vi "Lab7_Spectrum_Analyzer.vi"() -> ()   [LabVIEW 2016]
uses:
  <vilib>/Analysis/4window.llb/windowTd.ctl
  <vilib>/DAQmx/read.llb/DAQmx Read (Analog Wfm 1Chan NSamp).vi
  <vilib>/DAQmx/create/channels.llb/DAQmx Create Channel (AI-Voltage-Basic).vi
  <vilib>/DAQmx/configure/timing.llb/DAQmx Timing (Sample Clock).vi
  <vilib>/DAQmx/miscellaneous.llb/DAQmx Fill In Error Info.vi
  <vilib>/measure/maspectr.llb/FFT Power Spectrum and PSD for 1 Chan.vi
  <vilib>/measure/NI_MAPro.lvlib
  <vilib>/measure/NI_MABase.lvlib
  <vilib>/Analysis/NI_AALPro.lvlib
panel:
  out "quantized signal":waveform(ext)(graph)
  in  "full scale":dbl
  in  "number of bits":i16
  out "RMS dBV":dbl
  out "RMS":dbl
  out "Peak to Peak":dbl
  in  "rate":dbl=1000.0 format="%0.2f"
  out "Signal":waveform(dbl)(graph)
  in  "averaging parameters":T1={"averaging mode"=enum."No averaging", "weighting mode"=enum."Exponential", "number of averages"=10} {"number of averages" min=1}
  in  "dB On (F)":bool
  in  "window":T2=1 items=["Rectangle"=0, "Hanning"=1, "Hamming"=2, "Blackman-Harris"=3, "Exact Blackman"=4, "Blackman"=5, "Flat Top"=6, "4 Term B-Harris "=7, "7 Term B-Harris"=8, "Low Sidelobe"=9, "Blackman Nuttall"=11, "Triangle"=30, "Bartlett-Hanning"=31, "Bohman"=32, "Parzen"=33, "Welch"=34, "Kaiser"=60, "Dolph-Chebyshev"=61, "Gaussian"=62]
  in  "stop":bool
  in  "number of samples per channel":i32=-1
  out "Spectrum":cluster{"f0":dbl, "df":dbl, "magnitude":dbl[]}(graph)
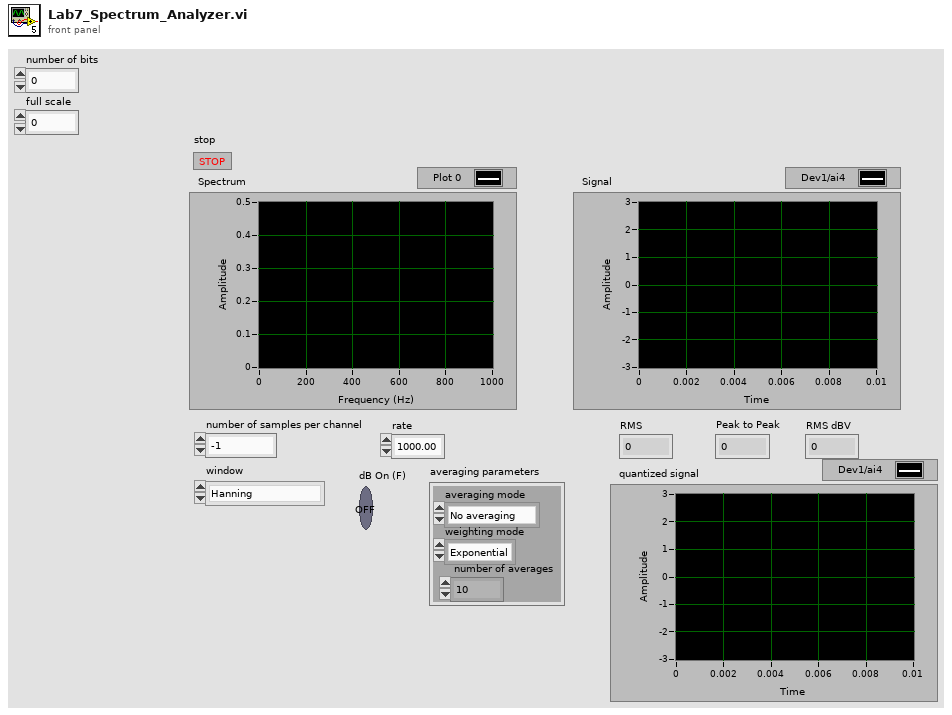
[diagram p1: front panel]
types:
  T1 = cluster{"averaging mode":enum16{"No averaging", "Vector averaging", "RMS averaging", "Peak hold"}, "weighting mode":enum16{"Linear", "Exponential"}, "number of averages":u32}
  T2 = typedef "NI_AALPro.lvlib/windowTd.ctl" = u32
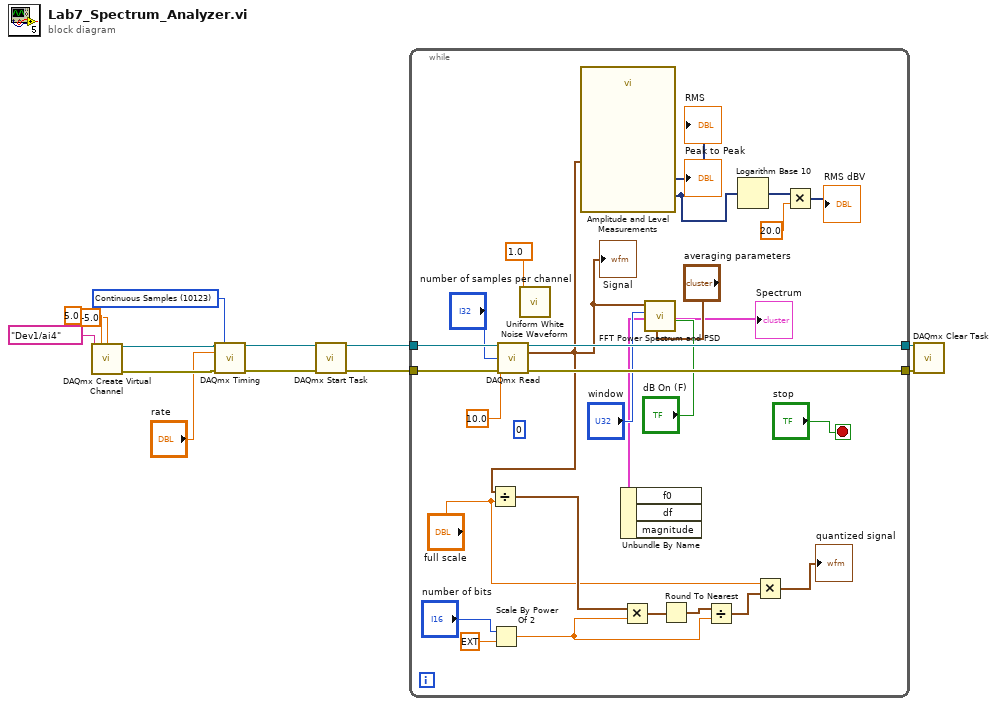
[diagram p0: block diagram]
diagram:
  w9 = 10123 items=["Finite Samples"=10178, "Continuous Samples"=10123, "Hardware Timed Single Point"=12522] ("sample mode")
  n1 = call-poly <vilib>:"DAQmx Create Virtual Channel.vi"("maximum value"=5.0, "minimum value"=-5.0, "physical channels"=tag "Dev1/ai4") -> ("task out"=w10:refnum<k21>, "error out"=w6:errorcluster)  [unwired: 11 in]
  n2 = call-poly <vilib>:"DAQmx Timing.vi"("task/channels in"=w10, "sample mode"=w9, "rate"="rate", "error in"=w6) -> ("task out"=w8:refnum<k21>, "error out"=w5:errorcluster)  [unwired: 10 in]
  n3 = call <vilib>:"DAQmx Start Task.vi"("task/channels in"=w8, "error in"=w5) -> ("task out"=w7:refnum<k21>, "error out"=w4:errorcluster)  [unwired: 12 in]
  n4 = while {
    tunnel: w7 -> [w40]
    tunnel: w4 -> [w37]
    tunnel: [w36] -> w3
    tunnel: [w35] -> w2
    stop <- "stop" stop-if-true
    (unwired) 0 ("seed")
    n5 = Scale By Power Of 2(n="number of bits", x=ext 1.0) -> (x*2^n=w19:ext)
    n6 = call-poly <vilib>:"DAQmx Read.vi"("task/channels in"=w40, "number of samples per channel"="number of samples per channel", "timeout"=10.0, "error in"=w37) -> ("task out"=w36:refnum<k21>, "data"=w22:waveform(dbl), "error out"=w35:errorcluster)  [unwired: 9 in]
    "Signal" <- w22
    n7 = Divide(x=w22, y="full scale") -> (x/y=w21:waveform(dbl))
    n8 = call <vilib>:"Uniform White Noise Waveform.vi"("amplitude"=1.0) -> ()  [unwired: 9 in, 2 out]
    n9 = call "Amplitude and Level Measurements"("Signals"=w22) -> ("RMS"=w29:dynamicdata, "Peak to Peak"=→"Peak to Peak":dynamicdata)  [unwired: 12 in, 1 out]
    "RMS" <- w29
    n10 = Multiply(x=w21, y=w19) -> (x*y=w20:waveform(ext))
    n11 = call-poly <vilib>:"FFT Power Spectrum and PSD.vi"("averaging parameters"="averaging parameters", "dB On (F)"="dB On (F)", "window"="window", "time signal"=w22) -> ("Power Spectrum / PSD"=w24:cluster{"f0":dbl, "df":dbl, "magnitude":dbl[]})  [unwired: 4 in, 3 out]
    "Spectrum" <- w24
    n12 = Unbundle By Name(w24) -> ()  [unwired: 3 out]
    n13 = Round To Nearest(number=w20) -> (nearest integer value=w18:waveform(ext))
    n14 = Divide(x=w18, y=w19) -> (x/y=w17:waveform(ext))
    n15 = Logarithm Base 10(1:w29) -> (0:w28:dynamicdata)
    n16 = Multiply(x="full scale", y=w17) -> (x*y=→"quantized signal":waveform(ext))
    n17 = Multiply(x=w28, y=20.0) -> (x*y=→"RMS dBV":dynamicdata)
  }
  n18 = call <vilib>:"DAQmx Clear Task.vi"("task in"=w3, "error in"=w2) -> ()  [unwired: 13 in, 1 out]
